vi "Read Measurement and Settling Cycles.vi"(0 "signal configuration":refnum<class "SV Function.lvclass">, 11 "error in (no error)":errorcluster) -> (4 "signal configuration":refnum<class "SV Function.lvclass">, 6 "measurement cycles":dbl=20.0, 8 "pre-measurement settling cycles":dbl, 10 "post-measurement settling cycles":dbl, 15 "error out":errorcluster)   [LabVIEW 2017, in "SV Function.lvclass"]
uses:
  <vilib>/addons/_NISVFA/_Generation/Signal Generation/SV Function/SV Function.lvclass
  <vilib>/addons/_NISVFA/_Generation/Signal Generation/SV Function/SV Function.lvclass/SV Function.ctl
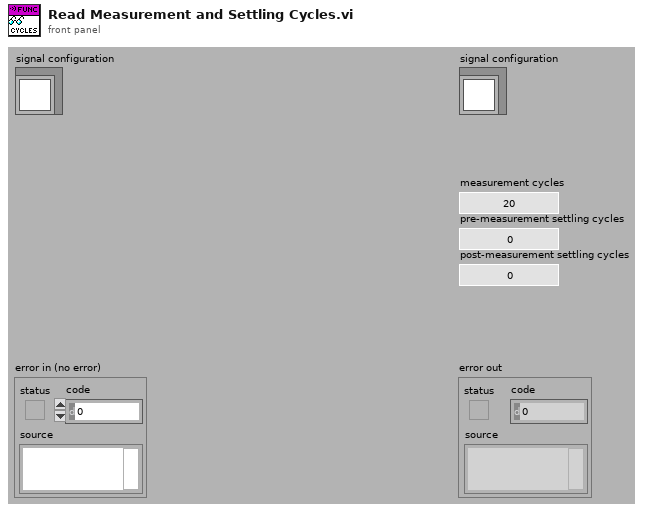
[diagram p1: front panel]
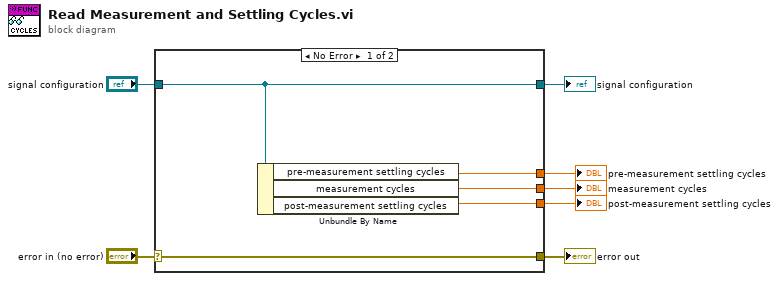
[diagram p0: block diagram]
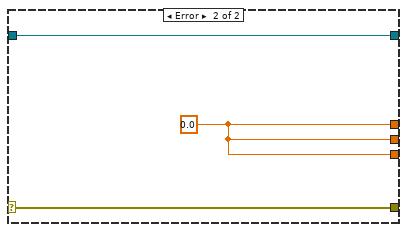
[diagram p2: hidden frame]
diagram:
  n1 = case shown="No Error" "error in (no error)" {
    selector: "error in (no error)" -> [w12 w14]
    tunnel: [w12 w14] -> w6
    tunnel: [w8 w15] -> w4
    tunnel: "signal configuration" -> [w8 w15]
    tunnel: [w11 w13] -> w3
    tunnel: [w10 w13] -> w2
    tunnel: [w9 w13] -> w1
    frame No Error {
      n2 = Unbundle By Name(w8) -> ("pre-measurement settling cycles"=w11:dbl, "measurement cycles"=w10:dbl, "post-measurement settling cycles"=w9:dbl)
    }
    frame Error {
      w13 = 0.0 ("measurement cycles")
    }
  }
  "error out" <- w6
  "signal configuration" <- w4
  "pre-measurement settling cycles" <- w3
  "measurement cycles" <- w2
  "post-measurement settling cycles" <- w1
